vi "音程計算.vi"(10 "音程":T2={"音級"=enum."一", "分類"=enum."完全"}, 11 "Note":T1={"音名"=enum."A", "度"=enum."0", "變音記號"=enum.""}) -> (2 "IsNoteExise?":bool, 3 "Note Out":T1={"音名"=enum."A", "度"=enum."0", "變音記號"=enum.""})   [LabVIEW 2015]
uses:
  Note.ctl
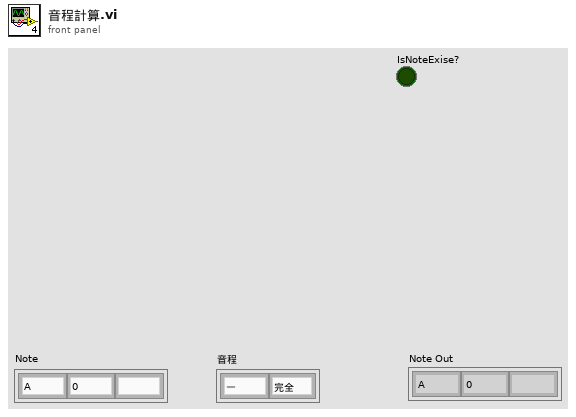
[diagram p1: front panel]
types:
  T1 = typedef "Note.ctl" = cluster{"音名":enum16{"C", "D", "E", "F", "G", "A", "B"}, "度":enum16{"0", "1", "2", "3", "4", "5", "6", "7", "8"}, "變音記號":enum16{"bb", "b", "", "#", "x"}}
  T2 = cluster{"音級":enum16{"一", "二", "三", "四", "き", "せ", "七", "八"}, "分類":enum16{"倍減", "減", "小", "完全", "大", "增", "倍增"}}
  T3 = enum16{"0", "1", "2", "3", "4", "5", "6", "7", "8"}
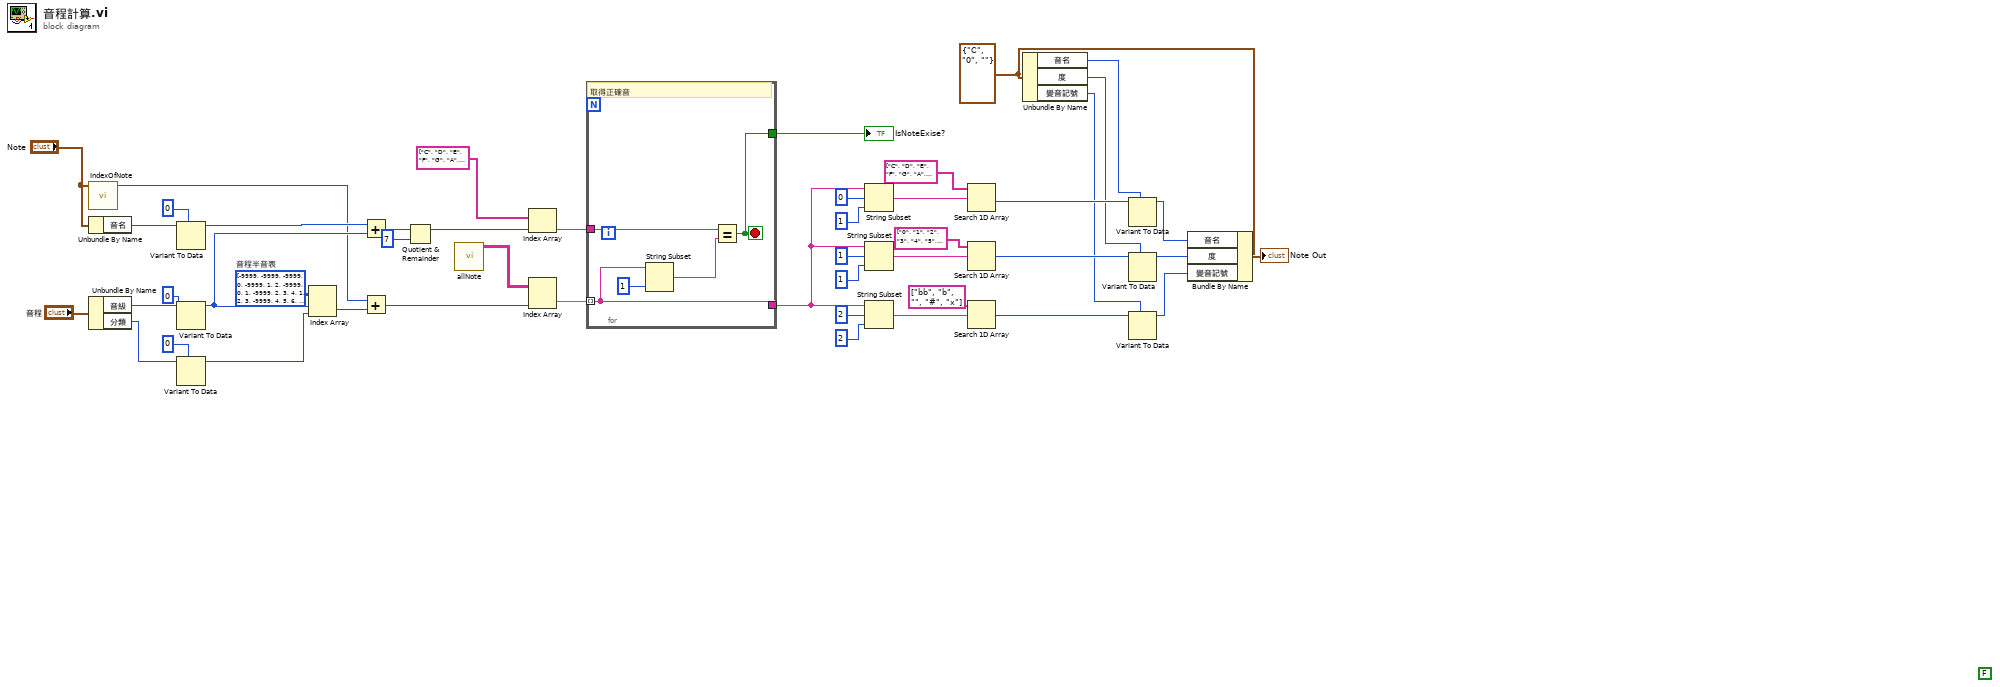
[diagram p0: block diagram]
diagram:
  w3 = T1 {"音名"=enum."C", "度"=enum."0", "變音記號"=enum.""} ("Note 2")
  (unwired) FALSE
  w42 = i32[][] [[-9999, -9999, -9999, 0, -9999, 1, 2], [-9999, 0, 1, -9999, 2, 3, 4], [1, 2, 3, -9999, 4, 5, 6], [3, 4, -9999, 5, -9999, 6, 7], [5, 6, -9999, 7, -9999, 8, 9], [6, 7, 8, -9999, 9, 10, 11], [8, 9, 10, -9999, 11, 12, 13], [10, 11, -9999, 12, -9999, 13, 14]]  # 音程半音表
  n1 = call "IndexOfNote.vi"("Note"="Note") -> ("index of note"=w12:i32)  [unwired: 9 in, 1 out]
  n2 = Unbundle By Name("Note") -> ("音名"=w33:enum16{"C", "D", "E", "F", "G", "A", "B"})
  n3 = Unbundle By Name("音程") -> ("音級"=w31:enum16{"一", "二", "三", "四", "き", "せ", "七", "八"}, "分類"=w30:enum16{"倍減", "減", "小", "完全", "大", "增", "倍增"})
  n4 = Variant To Data(type=0 ("y"), Variant=w33) -> (data=w35:i32)  [unwired: 1 in, 1 out]
  n5 = Variant To Data(type=0 ("y"), Variant=w31) -> (data=w38:i32)  [unwired: 1 in, 1 out]
  n6 = Variant To Data(type=0 ("y"), Variant=w30) -> (data=w39:i32)  [unwired: 1 in, 1 out]
  n7 = Index Array(array=w42, index (row)=w38, index (col)=w39) -> (element=w41:i32)
  n8 = Add(x=w35, y=w38) -> (x+y=w46:i32)
  n9 = Add(x=w12, y=w41) -> (x+y=w43:i32)
  n10 = Quotient & Remainder(x=w46, y=7) -> (x-y*floor(x/y)=w44:i32)  [unwired: 1 out]
  n11 = call "allNote.vi"() -> ("Allnote"=w11:string[][])  [unwired: 10 in, 1 out]
  n12 = Index Array(array=string[] ["C", "D", "E", "F", "G", "A", "B"], index=w44) -> (element=w45:string)
  n13 = Index Array(array=w11, index (col)=w43) -> (element=w47:string[])  [unwired: 1 in]
  n14 = for {
    tunnel: w47 -> [w49] mode=indexing
    tunnel: w45 -> [w51]
    tunnel: [w49] -> w23
    tunnel: [w48] -> w10
    stop <- w48 stop-if-true
    # "取得正確音"
    n15 = String Subset(string=w49, length (rest)=1 ("length (rest)")) -> (substring=w50:string)  [unwired: 1 in]
    n16 = Equal?(x=w51, y=w50) -> (x = y?=w48:bool)
  }
  "IsNoteExise?" <- w10
  n17 = String Subset(string=w23, offset (0)=0, length (rest)=1 ("length (rest)")) -> (substring=w15:string)
  n18 = String Subset(string=w23, offset (0)=1, length (rest)=1 ("length (rest)")) -> (substring=w14:string)
  n19 = String Subset(string=w23, offset (0)=2, length (rest)=2 ("length (rest)")) -> (substring=w20:string)
  n20 = Search 1D Array(1D array=string[] ["C", "D", "E", "F", "G", "A", "B"], element=w15) -> (index of element=w17:i32)  [unwired: 1 in]
  n21 = Search 1D Array(1D array=string[] ["0", "1", "2", "3", "4", "5", "6", "7", "8"], element=w14) -> (index of element=w18:i32)  [unwired: 1 in]
  n22 = Search 1D Array(1D array=string[] ["bb", "b", "", "#", "x"], element=w20) -> (index of element=w19:i32)  [unwired: 1 in]
  n23 = Unbundle By Name(w3) -> ("音名"=w6:enum16{"C", "D", "E", "F", "G", "A", "B"}, "度"=w5:T3, "變音記號"=w4:enum16{"bb", "b", "", "#", "x"})
  n24 = Variant To Data(type=w6, Variant=w17) -> (data=w2:enum16{"C", "D", "E", "F", "G", "A", "B"})  [unwired: 1 in, 1 out]
  n25 = Variant To Data(type=w5, Variant=w18) -> (data=w1:T3)  [unwired: 1 in, 1 out]
  n26 = Variant To Data(type=w4, Variant=w19) -> (data=w16:enum16{"bb", "b", "", "#", "x"})  [unwired: 1 in, 1 out]
  n27 = Bundle By Name(cluster=w3, "音名"=w2, "度"=w1, "變音記號"=w16) -> (→"Note Out":T1)
